vi "Run.vi"(8 "error in (no error)":errorcluster, 10 "Buffer Size":u64=2048, 11 "Mixer in":refnum<class "Mixer.lvclass">) -> (0 "error out":errorcluster)   [LabVIEW 2020, in "G-Audio.lvlib" / "Mixer.lvclass"]
uses:
  Mixer.lvclass
  Mixer.lvclass/Mixer.ctl
  6b6e21db-26d8-44fc-bcc7-090b1c1e96ee.vi
  Private/Result To Error.vi
  6b6e21db-26d8-44fc-bcc7-090b1c1e96ee.vi/4dfb5711-8d81-45a3-b3db-a84d40650863.vi
  6b6e21db-26d8-44fc-bcc7-090b1c1e96ee.vi/c8869513-30c6-44f2-a2d3-73232fe63870.vi
  Private/Audio Device Refnum To Value.vi
  6b6e21db-26d8-44fc-bcc7-090b1c1e96ee.vi/4dfb5711-8d81-45a3-b3db-a84d40650863.vi/53d6f456-6d93-41d3-8485-27023fbbbc96.vi
  6b6e21db-26d8-44fc-bcc7-090b1c1e96ee.vi/c8869513-30c6-44f2-a2d3-73232fe63870.vi/53d6f456-6d93-41d3-8485-27023fbbbc96.vi
  <vilib>/Utility/Data Type/Get Numeric Information.vi
  <vilib>/Utility/error.llb/Error Cluster From Error Code.vi
  Channel/Channel.lvclass
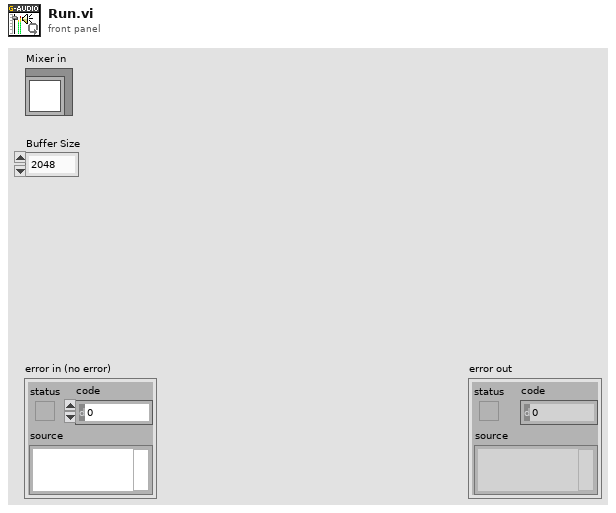
[diagram p1: front panel]
types:
  T1 = typedef "G-Audio.lvlib/Audio Device Refnum.ctl" = refnum<file>
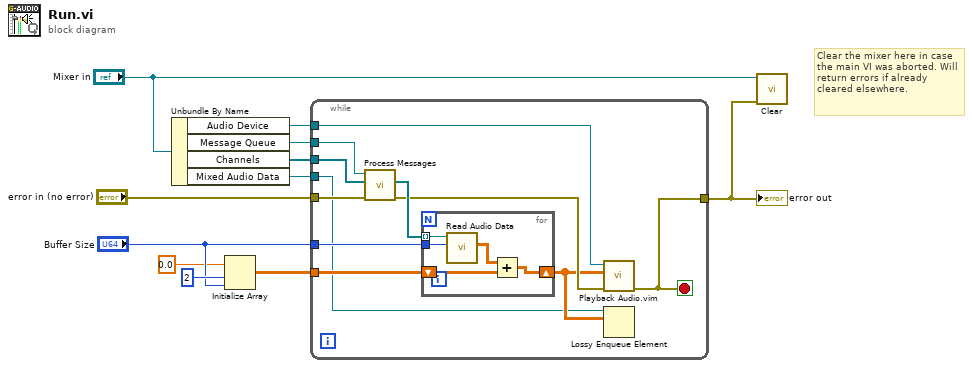
[diagram p0: block diagram]
diagram:
  # "Clear the mixer here in case the main VI was aborted. Will return errors if already cleared elsewhere."
  n1 = Unbundle By Name("Mixer in") -> ("Audio Device"=w11:T1, "Message Queue"=w5:refnum<queue>, "Channels"=w10:refnum<data-value>[], "Mixed Audio Data"=w1:refnum<queue>)
  n2 = Initialize Array(0.0 ("element"), u64 2 ("dimension size"), "Buffer Size") -> (w8:dbl[][])
  n3 = while {
    tunnel: w11 -> [w22]
    tunnel: w10 -> [w18]
    tunnel: w8 -> [w21]
    tunnel: "Buffer Size" -> [w20]
    tunnel: w5 -> [w19]
    tunnel: "error in (no error)" -> [w16]
    tunnel: [w14] -> w2
    tunnel: w1 -> [w12]
    stop <- w14 stop-if-true
    n4 = call "Process Messages.vi"("error in (no error)"=w16, "Channels in"=w18, "Message Queue"=w19) -> ("error out"=w15:errorcluster, "Channels out"=w17:refnum<data-value>[])  [unwired: 7 in]
    n5 = for {
      tunnel: w17 -> [w23] mode=indexing
      shift-right: [w27] -> w13
      shift-left: w21 -> [w26]
      tunnel: w20 -> [w24]
      n6 = call "Read Audio Data.vi"("Frames"=w24, "Channel in"=w23) -> ("Audio Data"=w25:dbl[][])  [unwired: 7 in, 2 out]
      n7 = Add(x=w25, y=w26) -> (x+y=w27:dbl[][])
    }
    n8 = call "Playback Audio.vim"("error in (no error)"=w15, "Audio Data"=w13, "Audio Device Refnum In"=w22) -> ("error out"=w14:errorcluster)  [unwired: 7 in, 1 out]
    n9 = Lossy Enqueue Element(queue=w12, element=w13) -> ()  [unwired: 1 in, 4 out]
  }
  "error out" <- w2
  n10 = call "Clear.vi"("error in (no error)"=w2, "Mixer in"="Mixer in") -> ()  [unwired: 9 in, 1 out]
